vi "Write Last Known State.vi"(7 "LC Type":T1, 8 "error in (no error)":errorcluster, 11 "FP-TC-Shared in":refnum<class "FP-TC-Shared.lvclass">) -> (0 "error out":errorcluster, 3 "FP-TC-Shared out":refnum<class "FP-TC-Shared.lvclass">)   [LabVIEW 2019, in "FP-TC-Shared.lvclass"]
uses:
  FP-TC-Shared.lvclass
  typedefs/LC Type--Enum.ctl
  FP-TC-Shared.lvclass/FP-TC-Shared.ctl
  <vilib>/Utility/config.llb/NI_LVConfig.lvlib
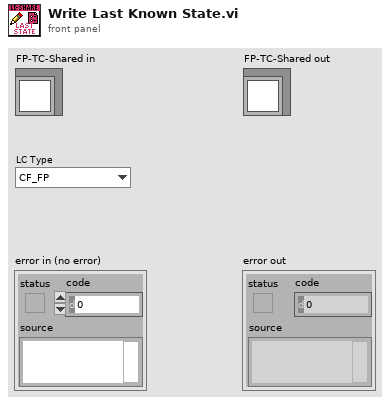
[diagram p1: front panel]
types:
  T1 = typedef "FP-TC-Shared.lvclass/LC Type--Enum.ctl" = enum16{"CF_FP", "CF_TC", "CF_TC_Z", "MNK_FP", "MNK_TC", "MNK_TC_Z", "unknown"}
  T2 = typedef "FP-TC-Shared.lvclass/Configuration--Cluster.ctl" = cluster{"Application":enum16{"TC", "FP"}, "LC Type":T1}
  T3 = typedef "NI_LVConfig.lvlib/Config Data RefNum.ctl" = refnum<k1>
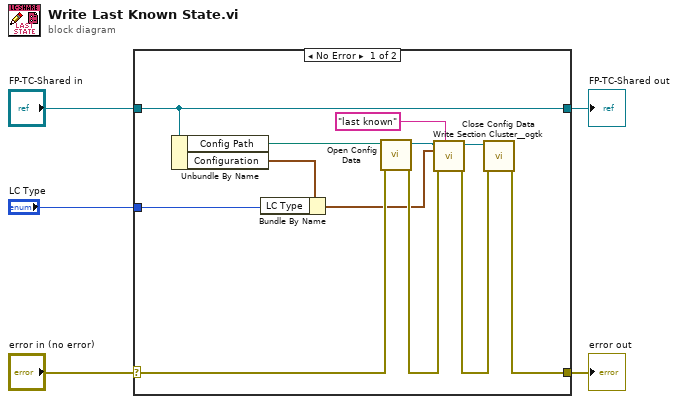
[diagram p0: block diagram]
diagram:
  n1 = case shown="No Error" "error in (no error)" {
    selector: "error in (no error)" -> [w12 w19]
    tunnel: [w9 w19] -> w4
    tunnel: [w17 w18] -> w2
    tunnel: "FP-TC-Shared in" -> [w17 w18]
    tunnel: "LC Type" -> [w6 _]
    frame No Error {
      n2 = Unbundle By Name(w17) -> ("Config Path"=w14:path, "Configuration"=w8:T2)
      n3 = Bundle By Name(cluster=w8, "LC Type"=w6) -> (w7:T2)
      n4 = call <vilib>:"Open Config Data.vi"("error in (no error)"=w12, "configuration file path"=w14) -> ("error out"=w11:errorcluster, "refnum"=w16:T3)  [unwired: 7 in, 1 out]
      n5 = call <userlib>:"Write Section Cluster__ogtk.vi"("section (optional)"="last known", "error in (no error)"=w11, "Section Formatted Cluster"=w7, "refnum"=w16) -> ("error out"=w10:errorcluster, "dup refnum"=w15:T3)  [unwired: 6 in]
      n6 = call <vilib>:"Close Config Data.vi"("error in (no error)"=w10, "refnum"=w15) -> ("error out"=w9:errorcluster)  [unwired: 8 in, 1 out]
    }
    frame Error {
    }
  }
  "error out" <- w4
  "FP-TC-Shared out" <- w2
